vi "SMC Setrate= Message.vi"(0 "Setrate":dbl format="%.2f") -> ()   [LabVIEW 2010]
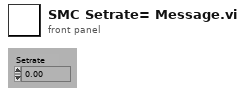
[diagram p1: front panel]
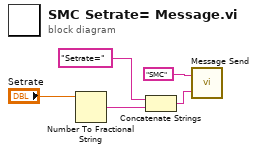
[diagram p0: block diagram]
diagram:
  n1 = Number To Fractional String(number="Setrate") -> (F-format string=w2:string)  [unwired: 3 in]
  n2 = Concatenate Strings("Setrate=" ("Message"), w2) -> (w5:string)
  n3 = call "Message Send.vi"("Message"=w5, "Destination"="SMC" ("Destination(s)")) -> ()
